vi "ToCombobox.vi"(8 "error in":errorcluster, 11 "Generic in":refnum<class "Generic.lvclass">) -> (0 "error out":errorcluster, 3 "Combobox out":refnum<class "Combobox.lvclass">)   [LabVIEW 2014, in "Combobox.lvclass"]
uses:
  Combobox.lvclass
  Generic/Generic.lvclass
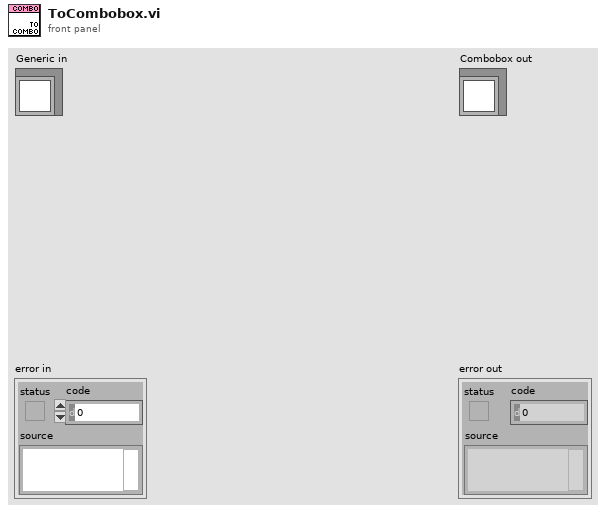
[diagram p1: front panel]
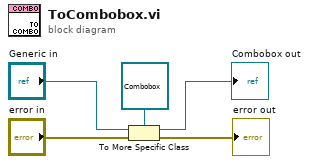
[diagram p0: block diagram]
diagram:
  n1 = To More Specific Class(target class=refnum<class "Combobox.lvclass"> refnum ("Combobox in"), reference="Generic in", error in="error in") -> (specific class reference=→"Combobox out":refnum<class "Combobox.lvclass">, error out=→"error out":errorcluster)
